vi "Divide Freq.vi"(7 "Divisor":i16, 9 "Self Clock":bool, 10 "Master Clock In":bool, 11 "Sync to Master?":bool) -> (2 "Step out":bool)   [LabVIEW 2014]
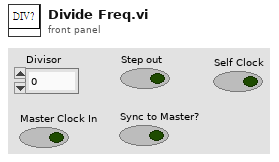
[diagram p1: front panel]
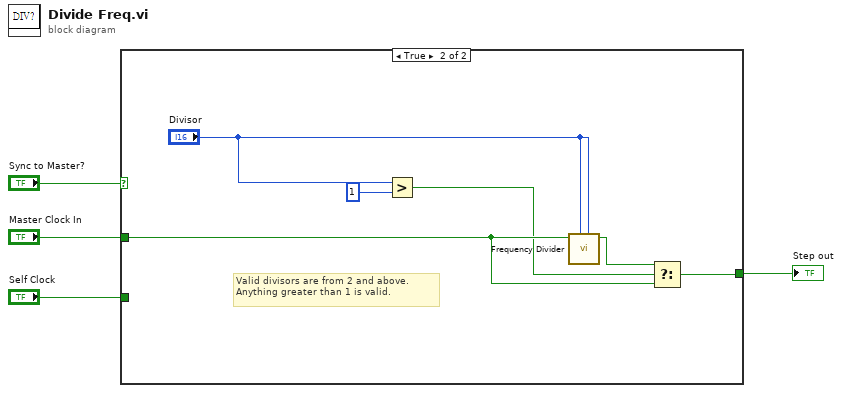
[diagram p0: block diagram]
diagram:
  n1 = case shown="True" "Sync to Master?" {
    tunnel: "Master Clock In" -> [_ w11]
    tunnel: [w5 w10] -> w3
    tunnel: "Self Clock" -> [w5 _]
    frame False {
      # "Passthrough"
    }
    frame True {
      # "Valid divisors are from 2 and above.\nAnything greater than 1 is valid."
      n2 = Greater?(x="Divisor", y=i16 1) -> (0:w8:bool)
      n3 = call "Frequency Divider.vi"("Highcounts"="Divisor", "Lowcounts"="Divisor", "Digital In"=w11) -> ("Digital Out"=w9:bool)  [unwired: 8 in]
      n4 = Select(t=w9, s=w8, f=w11) -> (s? t:f=w10:bool)
    }
  }
  "Step out" <- w3
